vi "Launch as Nested (Group).vi"(8 "error in (no error)":errorcluster, 9 "Group Config":refnum<class "Group.lvclass">, 10 "DataProcessor Config":refnum<class "Config Element.lvclass">, 11 "Parent Task in":refnum<class "Task.lvclass">) -> (0 "error out":errorcluster, 2 "API":refnum<class "DataHandlerAPI.lvclass">, 3 "Parent Task":refnum<class "Task.lvclass">)   [LabVIEW 2020, in "VolatusData.lvlib" / "DataProcessor.lvclass"]
uses:
  DataProcessor.lvclass
  DataHandlerAPI/DataHandlerAPI.lvclass
  C:/dev/lv20CE/relink/lv-volatus/Volatus/API/API.lvclass
  Volatus/Task/Task.lvclass
  VolatusConfig/Group/Group.lvclass
  lv-cdm/CDM-Config/Config Element/Config Element.lvclass
  C:/dev/lv20CE/relink/lv-volatus/Volatus/Task/Task.lvclass
  C:/dev/lv20CE/relink/lv-volatus/VolatusData/DataHandlerTask/DataHandlerTask.lvclass
  DataProcessor.lvclass/DataProcessor.ctl
  Volatus/Task/Task.lvclass/Task.ctl
  Volatus/VolatusAPI/VolatusAPI.lvclass/VolatusAPI.ctl
  Volatus/Event API/EventAPI.lvclass/EventAPI.ctl
  Volatus/EventHandler Messages/Handle Event Msg/Handle Event Msg.lvclass/Handle Event Msg.ctl
  <vilib>/ActorFramework/Message Enqueuer/Message Enqueuer.lvclass/Message Enqueuer.ctl
  Volatus/Event API/Report Event.vi
  Volatus/EventHandler Messages/Handle Event Msg/Send Handle Event.vi
  <vilib>/ActorFramework/Message Enqueuer/Enqueue.vi
  Volatus/EventHandler Messages/Handle Event Msg/Handle Event Msg.lvclass
  C:/Program Files (x86)/National Instruments/LabVIEW 2020/vi.lib/ActorFramework/Message/Message.lvclass
  <vilib>/ActorFramework/Message Priority Queue/Priority Enqueue.vi
  DataHandlerTask/DataHandlerTask.lvclass
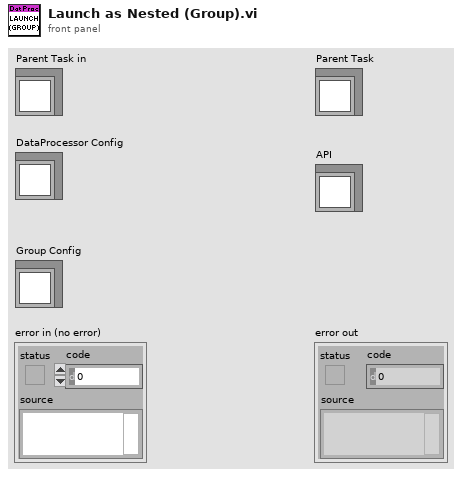
[diagram p1: front panel]
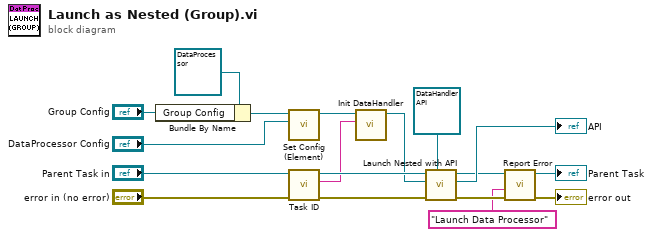
[diagram p0: block diagram]
diagram:
  n1 = Bundle By Name(cluster=refnum<class "DataProcessor.lvclass"> refnum ("Volatus:DataProcessor.lvclass"), "Group Config"="Group Config") -> (w5:refnum<class "DataProcessor.lvclass">)
  n2 = call "Set Config (Element).vi"("Config Element"="DataProcessor Config", "Task in"=w5) -> ("Task out"=w7:refnum<class "DataProcessor.lvclass">)  [unwired: 8 in, 1 out]
  n3 = call-dynamic "Task ID.vi"("error in (no error)"="error in (no error)", "Task in"="Parent Task in") -> ("error out"=w13:errorcluster, "Task ID"=w10:string, "Task out"=w15:refnum<class "Task.lvclass">)  [unwired: 7 in]
  n4 = call "Init DataHandler.vi"("Parent Name"=w10, "DataHandlerTask in"=w7) -> ("DataHandlerTask out"=w11:refnum<class "DataProcessor.lvclass">)  [unwired: 8 in, 1 out]
  n5 = call "Launch Nested with API.vi"("API Type"=refnum<class "DataHandlerAPI.lvclass"> refnum ("Volatus:DataHandlerAPI"), "error in (no error)"=w13, "Nested Task"=w11, "Task in"=w15) -> ("error out"=w18:errorcluster, "API"=→"API":refnum<class "DataHandlerAPI.lvclass">, "Task out"=w3:refnum<class "Task.lvclass">)  [unwired: 5 in]
  n6 = call "Report Error.vi"("error in (no error)"=w18, "Message"="Launch Data Processor", "Task in"=w3) -> ("error out"=→"error out":errorcluster, "Task out"=→"Parent Task":refnum<class "Task.lvclass">)  [unwired: 7 in]
